vi "Client_GetHelloClassique.vi"() -> ()   [LabVIEW 2020]
uses:
  <vilib>/httpClient/LabVIEWHTTPClient.lvlib
panel:
  out "error out":errorcluster
  out "body":string
  out "headers":string
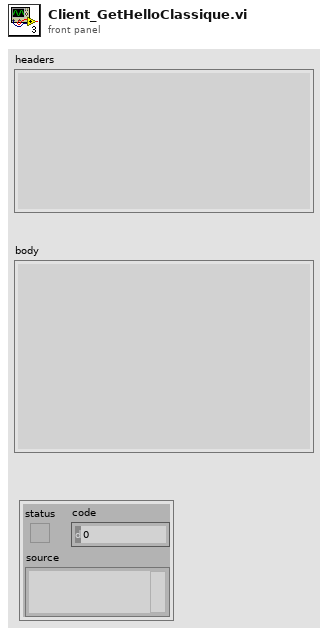
[diagram p1: front panel]
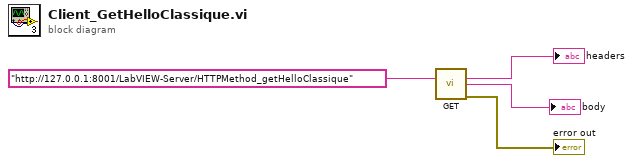
[diagram p0: block diagram]
diagram:
  n1 = call <vilib>:"GET.vi"("url"="http://127.0.0.1:8001/LabVIEW-Server/HTTPMethod_getHelloClassique") -> ("headers"=→"headers":string, "body"=→"body":string, "error out"=→"error out":errorcluster)  [unwired: 11 in, 1 out]
